vi "Close Variable Connections.vi"(11 "Variable References 2":T1) -> ()   [LabVIEW 2017]
uses:
  controls/CPU Loads.ctl
  controls/FPGA State.ctl
  <vilib>/vision/Image Controls.llb/IMAQ Image.ctl
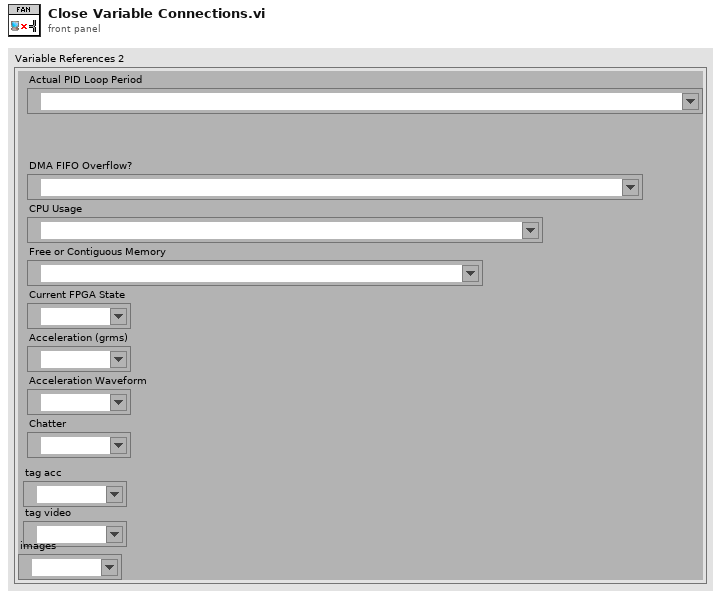
[diagram p1: front panel]
types:
  T1 = cluster{"Actual PID Loop Period":refnum<k21>, "DMA FIFO Overflow?":refnum<k21>, "CPU Usage":refnum<k21>, "Free or Contiguous Memory":refnum<k21>, "Current FPGA State":refnum<k21>, "Acceleration (grms)":refnum<k21>, "Acceleration Waveform":refnum<k21>, "Chatter":refnum<k21>, "tag acc":refnum<k21>, "tag video":refnum<k21>, "images":refnum<k21>}
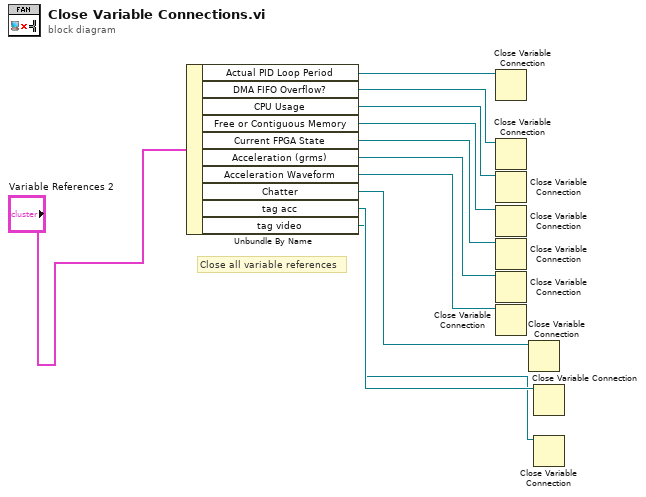
[diagram p0: block diagram]
diagram:
  # "Close all variable references"
  n1 = Unbundle By Name("Variable References 2") -> ("Actual PID Loop Period"=w8:refnum<k21>, "DMA FIFO Overflow?"=w7:refnum<k21>, "CPU Usage"=w6:refnum<k21>, "Free or Contiguous Memory"=w9:refnum<k21>, "Current FPGA State"=w10:refnum<k21>, "Acceleration (grms)"=w11:refnum<k21>, "Acceleration Waveform"=w5:refnum<k21>, "Chatter"=w4:refnum<k21>, "tag acc"=w3:refnum<k21>, "tag video"=w1:refnum<k21>)
  n2 = Close Variable Connection(11:w8) -> ()  [unwired: 1 in, 1 out]
  n3 = Close Variable Connection(11:w7) -> ()  [unwired: 1 in, 1 out]
  n4 = Close Variable Connection(11:w6) -> ()  [unwired: 1 in, 1 out]
  n5 = Close Variable Connection(11:w9) -> ()  [unwired: 1 in, 1 out]
  n6 = Close Variable Connection(11:w10) -> ()  [unwired: 1 in, 1 out]
  n7 = Close Variable Connection(11:w11) -> ()  [unwired: 1 in, 1 out]
  n8 = Close Variable Connection(11:w5) -> ()  [unwired: 1 in, 1 out]
  n9 = Close Variable Connection(11:w4) -> ()  [unwired: 1 in, 1 out]
  n10 = Close Variable Connection(11:w3) -> ()  [unwired: 1 in, 1 out]
  n11 = Close Variable Connection(11:w1) -> ()  [unwired: 1 in, 1 out]
